vi "Project - Ehsan Misaghi, Amir Hossein Jamali.vi"() -> ()   [LabVIEW 2012]
uses:
  <vilib>/Platform/TimedLoop/XDataNode/timing_clust.ctl
  <vilib>/Platform/TimedLoop/XDataNode/nitl_modes.ctl
  <vilib>/Platform/TimedLoop/XDataNode/wakeup.ctl
  <vilib>/platform/TimedLoop/XDataNode/XDataNode.xnode
  <vilib>/Platform/TimedLoop/XDataNode/XDNodeRunTimeDep.lvlib
  <vilib>/ptbypt/NI_PtbyPt.lvlib
panel:
  in  "Pause/Resume":bool
  out "F12-15":cluster{"Y":dbl[], "Y":dbl[]}[](graph)
  out "F8-12":cluster{"Y":dbl[], "Y":dbl[]}[](graph)
  out "F4-8":cluster{"Y":dbl[], "Y":dbl[]}[](graph)
  out "F0.5-4":cluster{"Y":dbl[], "Y":dbl[]}[](graph)
  out "Output":cluster{"Y":dbl[], "Y":dbl[]}[](graph)
  out "Time":i32
  out "Input":cluster{"Y":dbl[], "Y":dbl[]}[](graph)
  in  "Start/Stop":bool
  out "Current":string
  out "Container":string
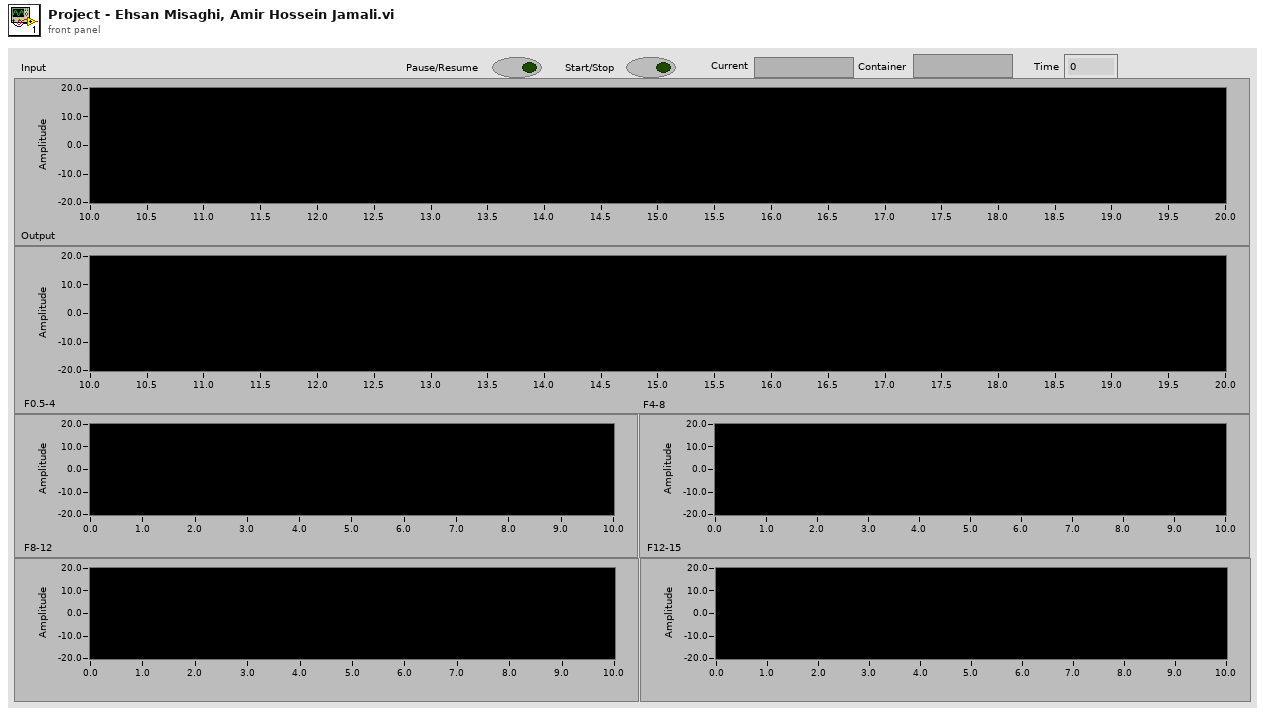
[diagram p1: front panel]
types:
  T1 = typedef "XDNodeRunTimeDep.lvlib/timing_clust.ctl" = cluster{"Expected End [f-1]":u64, "Actual End [f-1]":u64, "Finished Late? [f-1]":bool, "Expected End [i-1]":u64, "Actual End [i-1]":u64, "Finished Late? [i-1]":bool, "Expected Start [i]":u64, "Actual Start [i]":u64, "Expected Start [f]":u64, "Actual Start [f]":u64, "Source Name":string, "Structure Name":string, "Period":i64, "Deadline":i64, "Offset":i64, "Start":i64, "Priority":i32, "Timeout":i32, "Mode":T2, "Wakeup Reason":T3, "Error":errorcluster, "Source Type":string, "Secondary Source Type":string, "Global End Time":u64, "Global Start Time":u64, "Frame Duration":u64, "Iteration Duration":u64, "Assigned CPU":i32, "I/O Scan Engine Mode":u32}
  T2 = typedef "XDNodeRunTimeDep.lvlib/nitl_modes.ctl" = enum32{"No Change", "Process missed periods, maintain original phase", "Discard missed periods, maintain original phase", "Process missed periods, ignore original phase", "Discard missed periods, ignore original phase"}
  T3 = typedef "XDNodeRunTimeDep.lvlib/wakeup.ctl" = enum32{"Normal", "Aborted", "Asynchronous wakeup", "Timing source error", "Timed loop error", "Timeout"}
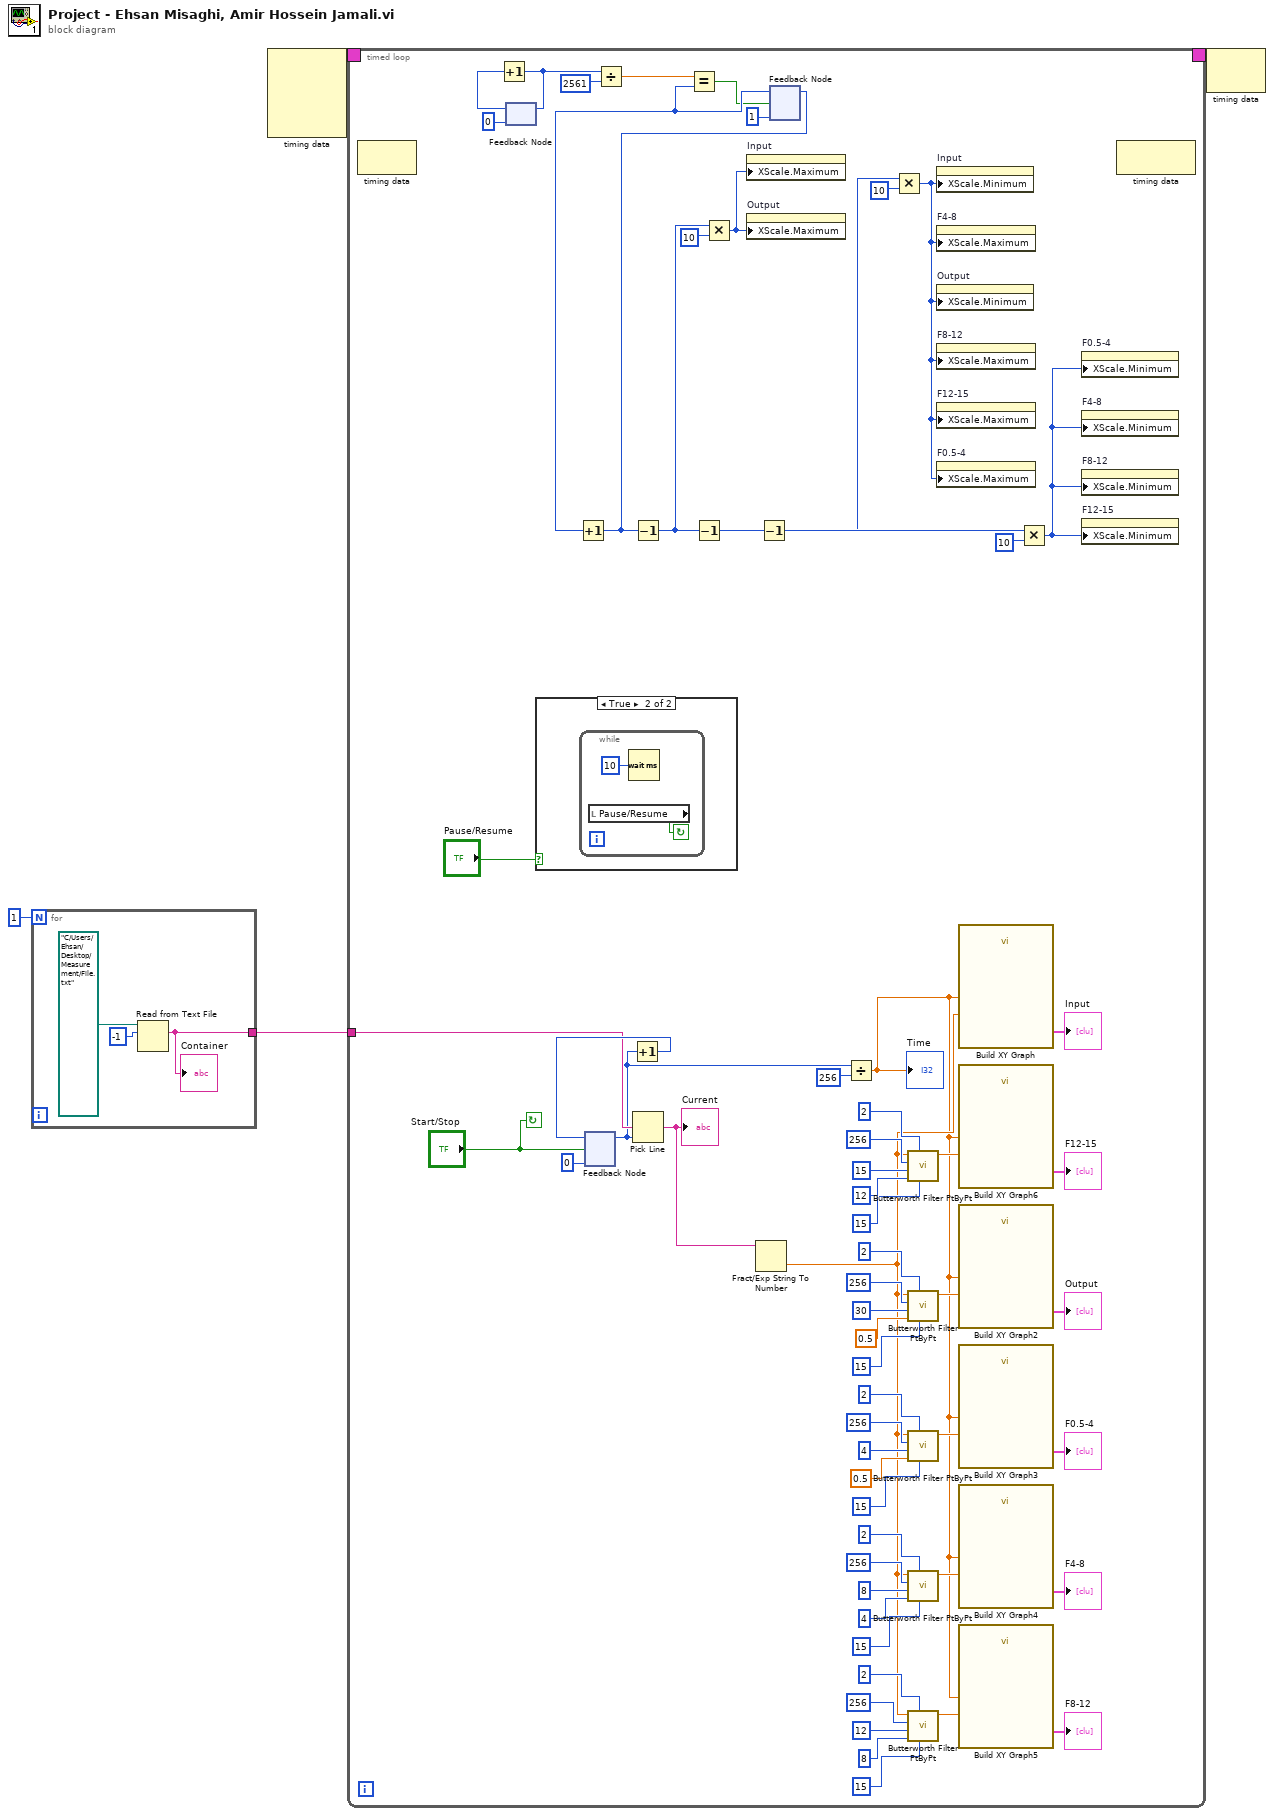
[diagram p0: block diagram]
diagram:
  n1 = for {
    N: 1 -> [_]
    tunnel: [w5] -> w1
    n2 = Read from Text File(file (use dialog)=path "C:/Users/Ehsan/Desktop/Measurement/File.txt", count=-1) -> (text=w5:string)  [unwired: 2 in, 3 out]
    "Container" <- w5
  }
  n3 = node-c288() -> (w4:T1)  [unwired: 4 in]
  n4 = timed-loop {
    timing: w4 -> [_]
    timing-out: [_] -> w3
    tunnel: w1 -> [w69]
    stop <- "Start/Stop" continue-if-true
    n5 = node-c288() -> ()  [unwired: 1 in, 1 out]
    n6 = feedback #1(0) -> (w64:i32)
    n7 = Increment(x=w64) -> (x+1=w61:i32)
    n8 = feedback-in #1(w61) -> ()
    n9 = case shown="True" "Pause/Resume" {
      frame False {
      }
      frame True {
        n10 = while {
          stop <- w73 continue-if-true
          n11 = local read "Pause/Resume"() -> (w73:bool)
          n12 = Wait (ms)(milliseconds to wait=u32 10) -> ()  [unwired: 1 out]
        }
      }
    }
    n13 = feedback #2(0) -> (w67:i32)
    n14 = Divide(x=w61, y=2561) -> (x/y=w62:dbl)
    n15 = Increment(x=w67) -> (x+1=w71:i32)
    n16 = feedback-in #2(w71, "Start/Stop") -> ()
    n17 = Pick Line(multi-line string=w69, line index=w67) -> (output string=w68:string)  [unwired: 1 in]
    "Current" <- w68
    n18 = Fract/Exp String To Number(string=w68) -> (number=w18:dbl)  [unwired: 3 in, 1 out]
    n19 = feedback #3(1) -> (w59:i32)
    n20 = Increment(x=w59) -> (x+1=w55:i32)
    n21 = Decrement(x=w55) -> (x-1=w54:i32)
    n22 = Equal?(x=w62, y=w59) -> (x = y?=w47:bool)
    n23 = Decrement(x=w54) -> (x-1=w13:i32)
    n24 = Multiply(x=w54, y=10) -> (x*y=w11:i32)
    n25 = property on="Input" class="XYGraph (strict)"("XScale.Maximum"=w11) -> ()  [unwired: 2 in, 2 out]
    n26 = property on="Output" class="XYGraph (strict)"("XScale.Maximum"=w11) -> ()  [unwired: 2 in, 2 out]
    n27 = Decrement(x=w13) -> (x-1=w15:i32)
    n28 = feedback-in #3(w55, w47) -> ()
    n29 = Divide(x=w67, y=256) -> (x/y=w17:dbl)
    "Time" <- w17
    n30 = Multiply(x=w13, y=10) -> (x*y=w10:i32)
    n31 = call <vilib>:"Butterworth Filter PtByPt.vi"("order"=15, "filter type"=2, "low cutoff freq: fl"=12, "high cutoff freq: fh"=15, "sampling freq: fs"=256, "x"=w18) -> ("Filtered x"=w24:dbl)  [unwired: 3 in, 1 out]
    n32 = call <vilib>:"Butterworth Filter PtByPt.vi"("order"=15, "filter type"=2, "low cutoff freq: fl"=0.5, "high cutoff freq: fh"=30, "sampling freq: fs"=256, "x"=w18) -> ("Filtered x"=w49:dbl)  [unwired: 3 in, 1 out]
    n33 = call <vilib>:"Butterworth Filter PtByPt.vi"("order"=15, "filter type"=2, "low cutoff freq: fl"=0.5, "high cutoff freq: fh"=4, "sampling freq: fs"=256, "x"=w18) -> ("Filtered x"=w42:dbl)  [unwired: 3 in, 1 out]
    n34 = call <vilib>:"Butterworth Filter PtByPt.vi"("order"=15, "filter type"=2, "low cutoff freq: fl"=4, "high cutoff freq: fh"=8, "sampling freq: fs"=256, "x"=w18) -> ("Filtered x"=w36:dbl)  [unwired: 3 in, 1 out]
    n35 = call <vilib>:"Butterworth Filter PtByPt.vi"("order"=15, "filter type"=2, "low cutoff freq: fl"=8, "high cutoff freq: fh"=12, "sampling freq: fs"=256, "x"=w18) -> ("Filtered x"=w30:dbl)  [unwired: 3 in, 1 out]
    n36 = property on="Input" class="XYGraph (strict)"("XScale.Minimum"=w10) -> ()  [unwired: 2 in, 2 out]
    n37 = property on="F4-8" class="XYGraph (strict)"("XScale.Maximum"=w10) -> ()  [unwired: 2 in, 2 out]
    n38 = property on="Output" class="XYGraph (strict)"("XScale.Minimum"=w10) -> ()  [unwired: 2 in, 2 out]
    n39 = property on="F8-12" class="XYGraph (strict)"("XScale.Maximum"=w10) -> ()  [unwired: 2 in, 2 out]
    n40 = property on="F12-15" class="XYGraph (strict)"("XScale.Maximum"=w10) -> ()  [unwired: 2 in, 2 out]
    n41 = property on="F0.5-4" class="XYGraph (strict)"("XScale.Maximum"=w10) -> ()  [unwired: 2 in, 2 out]
    n42 = call "Build XY Graph"("Y Input"=w18, "X Input"=w17) -> ("XY Graph"=→"Input":cluster{"Y":dbl[], "Y":dbl[]}[])  [unwired: 3 in, 6 out]
    n43 = call "Build XY Graph6"("Y Input"=w24, "X Input"=w17) -> ("XY Graph"=→"F12-15":cluster{"Y":dbl[], "Y":dbl[]}[])  [unwired: 3 in, 6 out]
    n44 = call "Build XY Graph2"("Y Input"=w49, "X Input"=w17) -> ("XY Graph"=→"Output":cluster{"Y":dbl[], "Y":dbl[]}[])  [unwired: 3 in, 6 out]
    n45 = call "Build XY Graph3"("Y Input"=w42, "X Input"=w17) -> ("XY Graph"=→"F0.5-4":cluster{"Y":dbl[], "Y":dbl[]}[])  [unwired: 3 in, 6 out]
    n46 = call "Build XY Graph4"("Y Input"=w36, "X Input"=w17) -> ("XY Graph"=→"F4-8":cluster{"Y":dbl[], "Y":dbl[]}[])  [unwired: 3 in, 6 out]
    n47 = call "Build XY Graph5"("Y Input"=w30, "X Input"=w17) -> ("XY Graph"=→"F8-12":cluster{"Y":dbl[], "Y":dbl[]}[])  [unwired: 3 in, 6 out]
    n48 = Multiply(x=w15, y=10) -> (x*y=w14:i32)
    n49 = property on="F0.5-4" class="XYGraph (strict)"("XScale.Minimum"=w14) -> ()  [unwired: 2 in, 2 out]
    n50 = property on="F4-8" class="XYGraph (strict)"("XScale.Minimum"=w14) -> ()  [unwired: 2 in, 2 out]
    n51 = property on="F8-12" class="XYGraph (strict)"("XScale.Minimum"=w14) -> ()  [unwired: 2 in, 2 out]
    n52 = property on="F12-15" class="XYGraph (strict)"("XScale.Minimum"=w14) -> ()  [unwired: 2 in, 2 out]
    n53 = node-c288() -> ()  [unwired: 1 in, 1 out]
  }
  n54 = node-c288(w3) -> ()  [unwired: 1 out]
